vi "Binary to Images(64-bit).vi"() -> ()   [LabVIEW 2013]
panel:
  out "Image/Sector Size(bytes)":i64
  in  "stop":bool
  out "Progress":u64(slide) max=5098 scale=0.0..1057.0
  out "Partial images in file?":bool
  out "# of Images":u32
  out "error IO":errorcluster
  out "Height":u32
  out "Width":u32
  in  "Created Image Path":path
  in  "Binary File":path
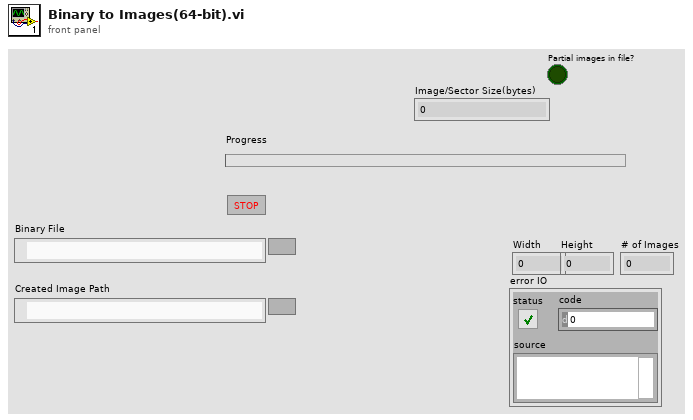
[diagram p1: front panel]
types:
  T1 = typedef "Image Type" = u32
  T2 = typedef "Mask ROI Cluster.ctl" = cluster{"left annulus":T3, "right annulus":T3, "Threshold Range":cluster{"Lower value":dbl, "Upper value":dbl}, "[Avg BG]":u8[], "Number of Sectors":u8, "Left ROI":T4, "Right ROI":T4, "Left Start Angle Duty Cycle":fxp<+,8,0>, "Left End Angle Duty Cycle":fxp<+,8,0>, "Right End Angle Duty Cycle":fxp<+,8,0>, "Right Start Angle Duty Cycle":fxp<+,8,0>, "[Sector ROIs]":T4[], "Consecutive Sector Threshold":u8}
  T3 = typedef "IMAQ Circle" = cluster{"Center X":i32, "Center Y":i32, "Inner Radius":i32, "Outer Radius":i32, "Start Angle":dbl, "End Angle":dbl}
  T4 = typedef "ROI Descriptor" = cluster{"Global Rectangle":i32[], "Contours":cluster{"ID":enum32{"External", "Internal"}, "Type":u32, "Coordinates":i32[]}[]}
  T5 = typedef "IMAQ Image.ctl" = refnum<image>
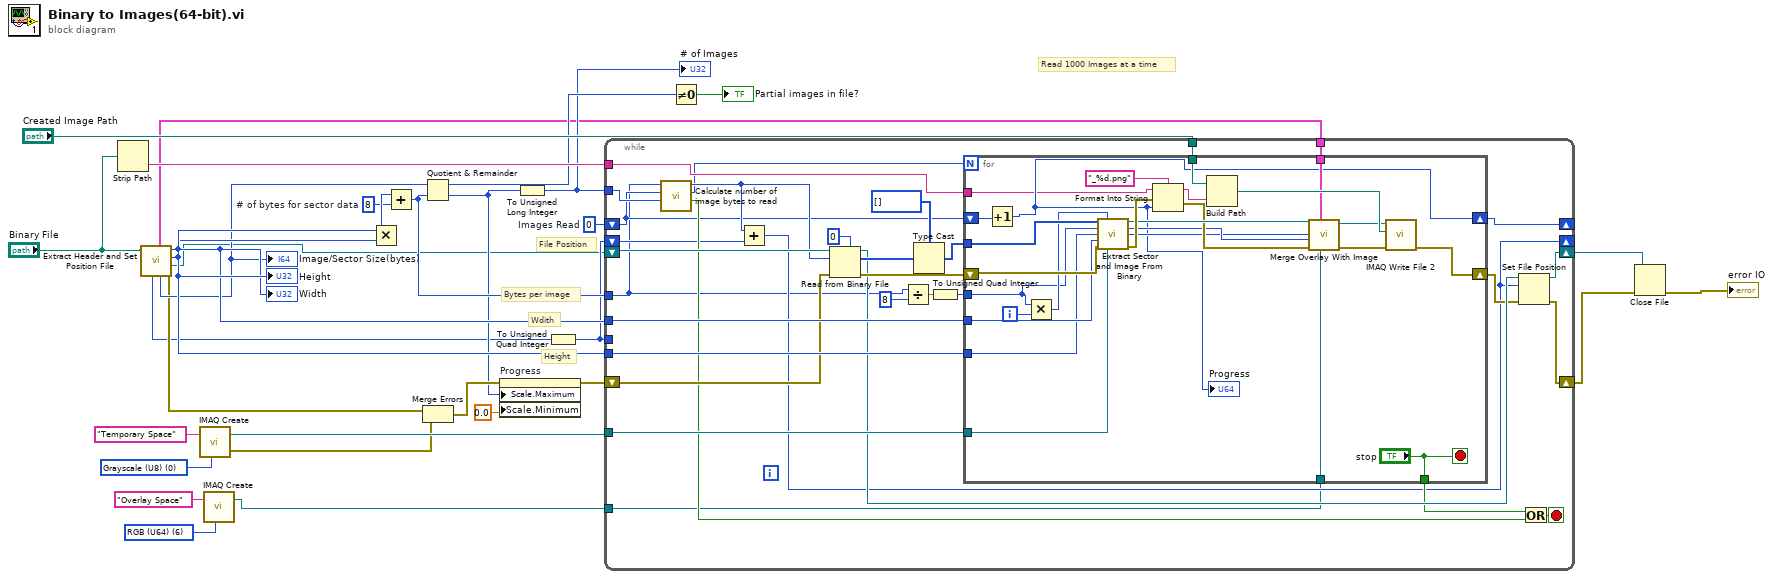
[diagram p0: block diagram]
diagram:
  w3 = T1 6 items=["Grayscale (U8)", "Grayscale (I16)", "Grayscale (SGL)", "Complex (CSG)", "RGB (U32)", "HSL (U32)", "RGB (U64)", "Grayscale (U16)"] ("Image Type")
  w10 = u32 0  # Images Read
  w16 = u32 8  # # of bytes for sector data
  w31 = T1 0 items=["Grayscale (U8)", "Grayscale (I16)", "Grayscale (SGL)", "Complex (CSG)", "RGB (U32)", "HSL (U32)", "RGB (U64)", "Grayscale (U16)"] ("Image Type")
  # "Height"
  # "Wdith"
  # "Bytes per image"
  # "File Position"
  # "Read 1000 Images at a time"
  n1 = Strip Path(path="Binary File") -> (name=w27:string)  [unwired: 1 out]
  n2 = call "Extract Header and Set Position File.vi"("Binary File"="Binary File") -> ("error out"=w11:errorcluster, "refnum out"=w4:refnum<file>, "Height"=w14:u32, "Width"=w13:u32, "Image/Sector Size(bytes)"=w12:i64, "Mask ROI Out"=w5:T2, "Header Size"=w7:i32)  [unwired: 4 in]
  "Width" <- w13
  "Height" <- w14
  "Image/Sector Size(bytes)" <- w12
  n3 = call "IMAQ Create"("Image Name"="Temporary Space", "Image Type"=w31) -> ("New Image"=w30:T5, "error out"=w29:errorcluster)  [unwired: 3 in]
  n4 = call "IMAQ Create"("Image Name"="Overlay Space", "Image Type"=w3) -> ("New Image"=w1:T5)  [unwired: 3 in, 1 out]
  n5 = Multiply(x=w14, y=w13) -> (x*y=w17:u32)
  n6 = Add(x=w17, y=w16) -> (x+y=w15:u32)
  n7 = Quotient & Remainder(x=w12, y=w15) -> (x-y*floor(x/y)=w23:i64, floor(x/y)=w9:i64)
  n8 = Merge Errors(w11, w29) -> (w21:errorcluster)
  n9 = property on="Progress" class="Slide (strict)"(error in=w21, "Scale.Maximum"=w9, "Scale.Minimum"=0.0 ("Data Entry Limits:Minimum")) -> (error out=w20:errorcluster)  [unwired: 1 in, 1 out]
  n10 = To Unsigned Long Integer(number=w9) -> (unsigned 32bit integer=w8:u32)
  "# of Images" <- w8
  n11 = To Unsigned Quad Integer(1:w7) -> (0:w6:u64)
  n12 = while {
    tunnel: w30 -> [w64]
    tunnel: "Created Image Path" -> [w63]
    tunnel: w27 -> [w62]
    tunnel: w13 -> [w61]
    tunnel: w14 -> [w60]
    shift-right: [w53] -> w25
    shift-left: w20 -> [w58]
    shift-right: [w51] -> w22
    shift-left: w4 -> [w59]
    tunnel: w15 -> [w37]
    tunnel: w6 -> [_]
    shift-right: [w42] -> _
    shift-left: w10 -> [w43]
    tunnel: w8 -> [w50]
    shift-right: [w39] -> _
    shift-left: w6 -> [w47]
    tunnel: w5 -> [w38]
    tunnel: w1 -> [w33]
    stop <- w48 stop-if-true
    n13 = call "Calculate number of image bytes to read.vi"("# of total images"=w50, "Total Images Read"=w43, "# of bytes per image"=w37) -> ("All Images Read?"=w49:bool, "# of Images Read"=w44:u32, "# of bytes to read"=w46:u64)  [unwired: 6 in]
    n14 = Add(x=w46, y=w47) -> (x+y=w39:u64)
    n15 = Read from Binary File(5:u8 0, 8:w58, 10:w46, 11:w59) -> (0:w57:errorcluster, 2:w55:u8[], 3:w52:refnum<file>)  [unwired: 2 in, 1 out]
    n16 = Divide(x=w37, y=u32 8) -> (x/y=w35:dbl)
    n17 = Type Cast(type=u64[] [], x=w55) -> (*(type *) &x=w45:u64[])
    n18 = To Unsigned Quad Integer(1:w35) -> (0:w34:u64)
    n19 = for {
      N: w44 -> [_]
      tunnel: w64 -> [w79]
      tunnel: w63 -> [w90]
      tunnel: w62 -> [w65]
      tunnel: w61 -> [w81]
      tunnel: w60 -> [w80]
      tunnel: w45 -> [w83]
      shift-right: [w68] -> w42
      shift-left: w43 -> [w77]
      shift-right: [w86] -> w41
      shift-left: w57 -> [w84]
      tunnel: ["stop"] -> w40
      tunnel: w38 -> [w71]
      tunnel: w34 -> [w67]
      tunnel: w33 -> [w66]
      i -> [w85]
      stop <- "stop" stop-if-true
      n20 = Increment(x=w77) -> (x+1=w68:u32)
      "Progress" <- w68
      n21 = Multiply(x=w67, y=w85) -> (x*y=w82:u64)
      n22 = call "Extract Sector and Image From Binary.vi"("Binary Data(u64)"=w83, "Start Index"=w82, "# of u64 per image"=w67, "Height"=w80, "Width"=w81, "error in (no error)"=w84, "Image Destination"=w79) -> ("Image Out"=w75:T5, "Left Sector"=w70:u16, "Right Sector"=w69:u16, "error out"=w78:errorcluster)  [unwired: 5 in]
      n23 = Format Into String(format string="_%d.png", initial string=w65, error in=w78, w68) -> (resulting string=w88:string, error out=w72:errorcluster)
      n24 = Build Path(base path=w90, name or relative path=w88) -> (appended path=w87:path)
      n25 = call "Merge Overlay With Image.vi"("Image In(Dst)"=w66, "ROI Cluster"=w71, "Error in"=w72, "Left Edge"=w70, "Right Edge"=w69, "Image In"=w75) -> ("error out"=w73:errorcluster, "Image Out"=w74:T5)  [unwired: 4 in]
      n26 = call-poly "IMAQ Write File 2"("error in (no error)"=w73, "File Path"=w87, "Image"=w74) -> ("error out"=w86:errorcluster)  [unwired: 7 in, 1 out]
    }
    n27 = Set File Position(offset (in bytes) (0)=w39, refnum=w52, error in=w41) -> (refnum out=w51:refnum<file>, error out=w53:errorcluster)  [unwired: 1 in]
    n28 = Or(x=w40, y=w49) -> (x .or. y?=w48:bool)
  }
  n29 = Not Equal To 0?(x=w23) -> (x != 0?=→"Partial images in file?":bool)
  n30 = Close File(refnum=w22, error in=w25) -> (error out=→"error IO":errorcluster)  [unwired: 1 out]
